vi "Update_String_client.vi"(1 "String":string, 2 "Ch Name":string) -> ()   [LabVIEW 2021]
uses:
  Sub VIs/ADAM Controls/Channel_State.ctl
  Sub VIs/ADAM Controls/Update_scan_value.ctl
  Sub VIs/ADAM Controls/Calib_type_ADAM.ctl
  Sub VIs/ADAM Controls/Module_type_ADAM.ctl
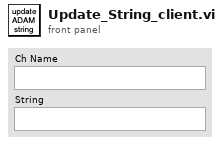
[diagram p1: front panel]
types:
  T1 = typedef "Module_type_ADAM.ctl" = string
  T2 = typedef "Calib_type_ADAM.ctl" = string
  T3 = typedef "Update_scan_value.ctl" = cluster{"Channel Name":string, "New Value":dbl, "!Auto_Off":bool}
  T4 = typedef "Channel_State.ctl" = enum16{"On", "Off", "Always On", "Always Off"}
  T5 = typedef "Ch_description_ADAM.ctl" = cluster{"Ch Name":string, "Type":T1, "Function":T6, "Ch State":T4, "Calibration type":T2, "A":dbl, "B":dbl, "C":dbl, "D":dbl, "Comments":string, "Address":T7, "String":string, "Duty":u16}
  T6 = typedef "Function_ADAM.ctl" = enum16{"Analogue Input", "Digital Input", "Event counter", "Event rate", "Analogue Output", "Digital Output", "Relay Output"}
  T7 = typedef "Address.ctl" = cluster{"Main":i32, "Ch.":i32, "Sub":i32, "Port Name":string}
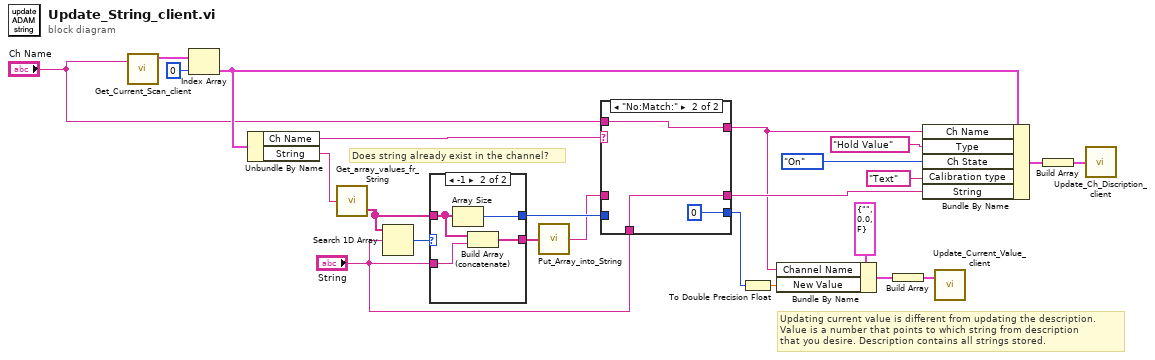
[diagram p0: block diagram]
diagram:
  # "Updating current value is different from updating the description.\nValue is a number that points to which string from description \nthat you desire. Description contains all strings stored."
  # "Does string already exist in the channel?"
  n1 = call "Get_Current_Scan_client.vi"("singleChannel"="Ch Name") -> ("Ch Description Array"=w24:T5[])  [unwired: 1 in, 3 out]
  n2 = Index Array(array=w24, index=0) -> (element=w4:T5)
  n3 = Unbundle By Name(w4) -> ("Ch Name"=w20:string, "String"=w18:string)
  n4 = call "Get_array_values_fr_String.vi"("String Value"=w18) -> ("String array"=w15:string[])  [unwired: 1 out]
  n5 = Search 1D Array(1D array=w15, element="String") -> (index of element=w16:i32)  [unwired: 1 in]
  n6 = case shown="-1" w16 {
    selector: w16 -> [w26 _]
    tunnel: [w26 w27] -> w17
    tunnel: [w25 w29] -> w14
    tunnel: w15 -> [w25 w28]
    tunnel: "String" -> [_ w30]
    frame Default {
    }
    frame -1 {
      n7 = Array Size(array=w28) -> (size(s)=w27:i32)
      n8 = Build Array (concatenate)(w28, w30) -> (w29:string[])
    }
  }
  n9 = call "Put_Array_into_String.vi"("String array"=w14) -> ("String Value"=w13:string)
  n10 = case shown="\"No:Match:\"" w20 {
    selector: w20 -> [w33 _]
    tunnel: [w33 w34] -> w7
    tunnel: "Ch Name" -> [_ w34]
    tunnel: [w32 0 ("index of element")] -> w8
    tunnel: w17 -> [w32 _]
    tunnel: [w31 w35] -> w12
    tunnel: w13 -> [w31 _]
    tunnel: "String" -> [_ w35]
    frame "", Default {
    }
    frame "No:Match:" {
    }
  }
  n11 = To Double Precision Float(number=w8) -> (double precision float=w9:dbl)
  n12 = Bundle By Name(cluster=T3 {"Channel Name"="", "New Value"=0.0, "!Auto_Off"=FALSE} ("Update Scan Value Cluster"), "Channel Name"=w7, "New Value"=w9) -> (w6:T3)
  n13 = Build Array(w6) -> (w5:T3[])
  n14 = Bundle By Name(cluster=w4, "Ch Name"=w7, "Type"=T1 "Hold Value", "Ch State"=Channel_State."On", "Calibration type"=T2 "Text", "String"=w12) -> (w23:T5)
  n15 = call "Update_Current_Value_client.vi"("Update array in"=w5) -> ()  [unwired: 1 in]
  n16 = Build Array(w23) -> (w22:T5[])
  n17 = call "Update_Ch_Discription_client.vi"("Channels to update In"=w22) -> ()  [unwired: 1 out]
